vi "Roller Motor Control.vi"(10 "RollerState":T1, 11 "RelayDevRef":T2={"DevStatus"={"status"=FALSE, "code"=0, "source"=""}, "Relay Channel"=enum."Invalid", "Digital Module"=enum."Digital Module 1", "Relay Direction"=enum."Both directions"}) -> ()   [LabVIEW 2013]
uses:
  <vilib>/Rock Robotics/WPI/Relay/WPI_RelayDevRef.ctl
  <vilib>/Rock Robotics/SystemInterfaces/DIO/FPGA_DIORelayChannel.ctl
  <vilib>/Rock Robotics/SystemInterfaces/Typedef/FPGA_TypedefDigitalModule.ctl
  <vilib>/Rock Robotics/WPI/Relay/WPI_RelayDirection.ctl
  Roller States.ctl
  <vilib>/Rock Robotics/WPI/Relay/WPI_RelayValue.ctl
panel:
  out "error out":errorcluster
  in  "error in (no error)":errorcluster
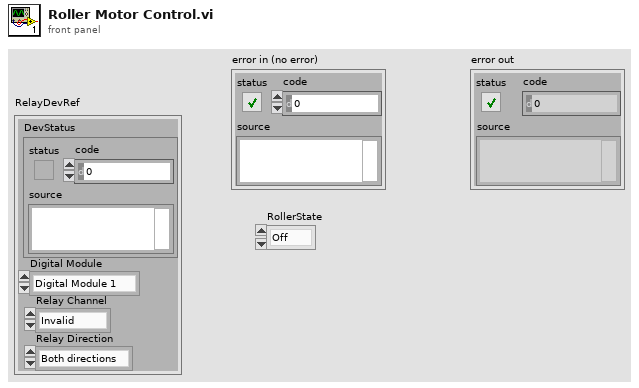
[diagram p1: front panel]
types:
  T1 = typedef "Roller States.ctl" = enum16{"Off", "Forward", "Reverse"}
  T2 = typedef "WPI_RelayDevRef.ctl" = cluster{"DevStatus":errorcluster, "Relay Channel":T3, "Digital Module":T4, "Relay Direction":T5}
  T3 = typedef "FPGA_DIORelayChannel.ctl" = enum8{"Relay 1", "Relay 2", "Relay 3", "Relay 4", "Relay 5", "Relay 6", "Relay 7", "Relay 8", "Invalid"}
  T4 = typedef "FPGA_TypedefDigitalModule.ctl" = enum16{"Digital Module 1", "Digital Module 2"}
  T5 = typedef "WPI_RelayDirection.ctl" = enum16{"Both directions", "Forward only", "Reverse only"}
  T6 = typedef "WPI_RelayValue.ctl" = enum16{"Off", "On", "Forward", "Reverse"}
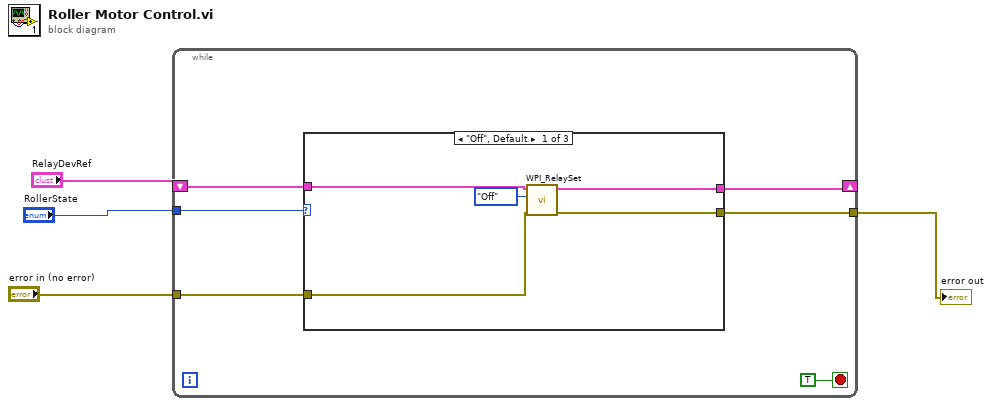
[diagram p0: block diagram]
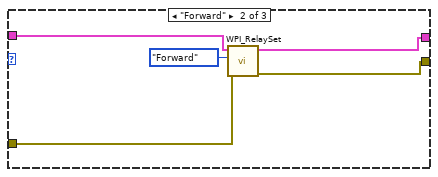
[diagram p2: hidden frame]
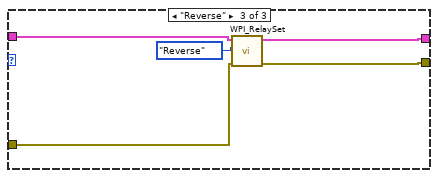
[diagram p3: hidden frame]
diagram:
  n1 = while {
    tunnel: "RollerState" -> [w10]
    shift-right: [w7] -> _
    shift-left: "RelayDevRef" -> [w8]
    tunnel: "error in (no error)" -> [w6]
    tunnel: [w5] -> w1
    stop <- TRUE stop-if-true
    n2 = case shown="\"Off\", Default" w10 {
      tunnel: w8 -> [w15 w20 w24]
      tunnel: [w14 w19 w23] -> w7
      tunnel: w6 -> [w12 w17 w22]
      tunnel: [w11 w16 w21] -> w5
      frame "Off", Default {
        n3 = call <vilib>:"WPI_RelaySet.vi"("error in (no error)"=w12, "RelayValue"=WPI_RelayValue."Off", "RelayDevRef"=w15) -> ("error out"=w11:errorcluster, "RelayDevRef"=w14:T2)  [unwired: 7 in]
      }
      frame "Forward" {
        n4 = call <vilib>:"WPI_RelaySet.vi"("error in (no error)"=w17, "RelayValue"=WPI_RelayValue."Forward", "RelayDevRef"=w20) -> ("error out"=w16:errorcluster, "RelayDevRef"=w19:T2)  [unwired: 7 in]
      }
      frame "Reverse" {
        n5 = call <vilib>:"WPI_RelaySet.vi"("error in (no error)"=w22, "RelayValue"=WPI_RelayValue."Reverse", "RelayDevRef"=w24) -> ("error out"=w21:errorcluster, "RelayDevRef"=w23:T2)  [unwired: 7 in]
      }
    }
  }
  "error out" <- w1
